vi "Wheel Set.vi"(9 "MotorControlDevRef":T2={"DeviceStatus"={"status"=FALSE, "code"=0, "source"=""}, "Type"=enum."PWM", "PWM"={"PWM Channel"=enum."Invalid", "DeadBand"={"Name"="", "maxPositivePwm"=0, "minPositivePwm"=0, "centerPwm"=0, "maxNegativePwm"=0, "minNegativePwm"=0, "angularRange"=0}}, "CAN"={"Device Number"=0, "Control Mode"=enum."Percent VBus", "Semaphore"=refnum, "Max Vout"=12.0, "TalonSRX Control Mode"=enum."Percent VBus"}, "Invert"=FALSE}, 10 "DevRef":string, 11 "Control Gains":T1={"Period (ms)"=20, "TBH Gain"=0.5, "Priority"=100, "PID gains"={"proportional gain (Kc)"=1.0, "integral time (Ti, min)"=0.01, "derivative time (Td, min)"=0.0}, "Stable (sec)"=20.0, "Range"=20.0} {"PID gains"."derivative time (Td, min)" format="%.3f"; "PID gains"."integral time (Ti, min)" format="%.3f"; "PID gains"."proportional gain (Kc)" format="%.3f"}) -> (0 "Error Out":errorcluster, 3 "Shooter Wheel DevRef Out":T9={"Shooter Config reference"=refnum, "Shooter Data"={"MotorControlDevRef"={"DeviceStatus"={"status"=FALSE, "code"=0, "source"=""}, "Type"=enum."PWM", "PWM"={"PWM Channel"=enum."Invalid", "DeadBand"={"Name"="", "maxPositivePwm"=0, "minPositivePwm"=0, "centerPwm"=0, "maxNegativePwm"=0, "minNegativePwm"=0, "angularRange"=0}}, "CAN"={"Device Number"=0, "Control Mode"=enum."Percent VBus", "Semaphore"=refnum, "Max Vout"=12.0, "TalonSRX Control Mode"=enum."Percent VBus"}, "Invert"=FALSE}, "Set Point"=refnum, "Actual"=refnum}})   [LabVIEW 2015, in "Wheel.lvlib"]
doc: "Help by FRC Team 836 - The RoboBees\n\nThis VI will set the desired Revolutions Per Minute (RPM) for a wheel."
uses:
  <userlib>/836-Library/Motion_Control/Shooter_Wheel/Wheel.lvlib
  <userlib>/836-Library/Motion_Control/Shooter_Wheel/WheelControl.ctl
  <userlib>/836-Library/Motion_Control/Shooter_Wheel/Config.ctl
  <userlib>/836-Library/Motion_Control/Shooter_Wheel/Data.ctl
  <vilib>/Rock Robotics/WPI/MotorControl/WPI_MotorControlDeviceRef.ctl
  <vilib>/Rock Robotics/WPI/MotorControl/WPI_MotorControlType.ctl
  <vilib>/Rock Robotics/SystemInterfaces/DIO/FPGA_DIOPWMChannel.ctl
  <vilib>/Rock Robotics/WPI/PWM/WPI_PWMDeadband.ctl
  <vilib>/Rock Robotics/WPI/CAN/Jaguar/SubVIs/WPI_CANJaguar_ControlMode.ctl
  <vilib>/Rock Robotics/WPI/CAN/TalonSRX/WPI_CANTalonSRX_APIControlMode.ctl
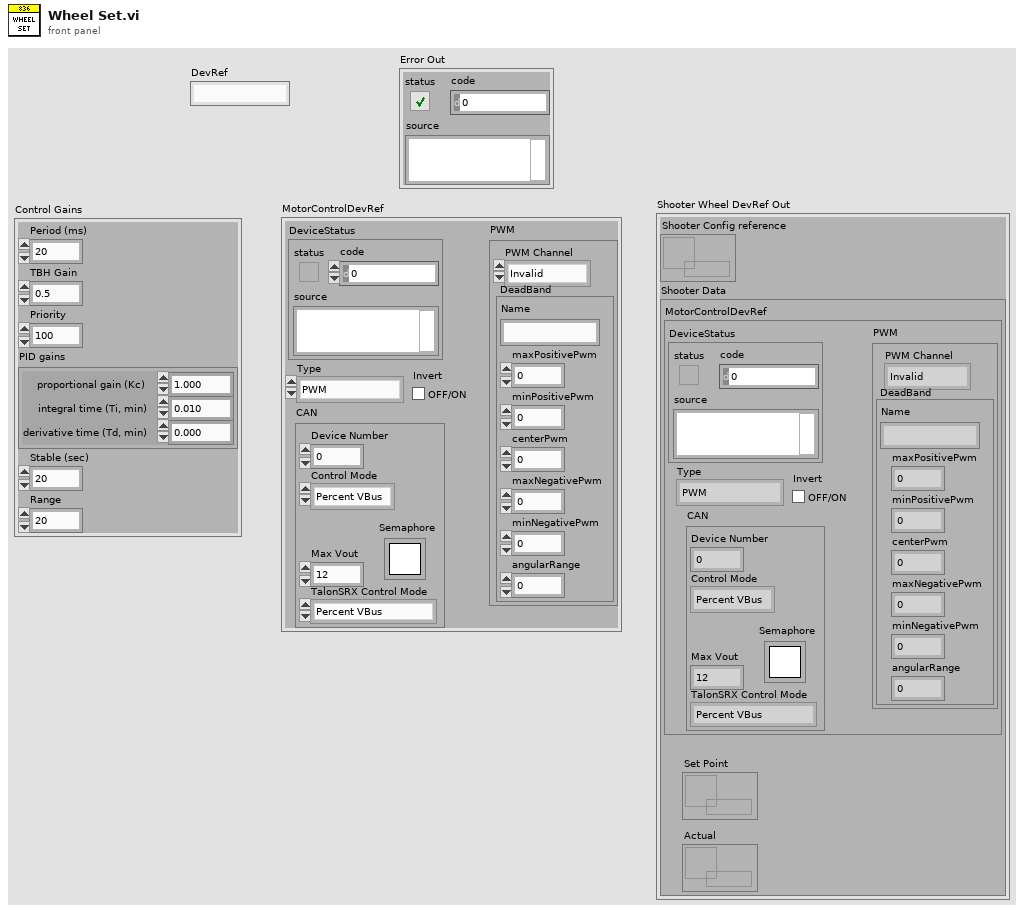
[diagram p1: front panel]
types:
  T1 = typedef "Wheel.lvlib/Config.ctl" = cluster{"Period (ms)":i64, "TBH Gain":dbl, "Priority":i32, "PID gains":cluster{"proportional gain (Kc)":dbl, "integral time (Ti, min)":dbl, "derivative time (Td, min)":dbl}, "Stable (sec)":dbl, "Range":dbl}
  T2 = typedef "WPI_MotorControlDeviceRef.ctl" = cluster{"DeviceStatus":errorcluster, "Type":T3, "PWM":cluster{"PWM Channel":T4, "DeadBand":T5}, "CAN":cluster{"Device Number":u8, "Control Mode":T6, "Semaphore":T7, "Max Vout":dbl, "TalonSRX Control Mode":T8}, "Invert":bool}
  T3 = typedef "WPI_MotorControlType.ctl" = enum16{"PWM", "CAN", "CANTalonSRX"}
  T4 = typedef "FPGA_DIOPWMChannel.ctl" = enum8{"PWM 0", "PWM 1", "PWM 2", "PWM 3", "PWM 4", "PWM 5", "PWM 6", "PWM 7", "PWM 8", "PWM 9", "PWM MXP 0", "PWM MXP 1", "PWM MXP 2", "PWM MXP 3", "PWM MXP 4", "PWM MXP 5", "PWM MXP 6", "PWM MXP 7", "PWM MXP 8", "PWM MXP 9", "Invalid"}
  T5 = typedef "WPI_PWMDeadband.ctl" = cluster{"Name":string, "maxPositivePwm":i32, "minPositivePwm":i32, "centerPwm":i32, "maxNegativePwm":i32, "minNegativePwm":i32, "angularRange":u16}
  T6 = typedef "WPI_CANJaguar_ControlMode.ctl" = enum8{"Percent VBus", "Current", "Speed", "Position", "Voltage"}
  T7 = typedef "Semaphore RefNum" = refnum<k1>
  T8 = typedef "WPI_CANTalonSRX_APIControlMode.ctl" = enum8{"Percent VBus", "Speed", "Position", "Slave", "Unchanged / Invalid", "Voltage Compensation", "Current", "Motion Profile"}
  T9 = typedef "Wheel.lvlib/WheelControl.ctl" = cluster{"Shooter Config reference":refnum<data-value>, "Shooter Data":T10}
  T10 = typedef "Wheel.lvlib/Data.ctl" = cluster{"MotorControlDevRef":T2, "Set Point":refnum<k33>, "Actual":refnum<k33>}
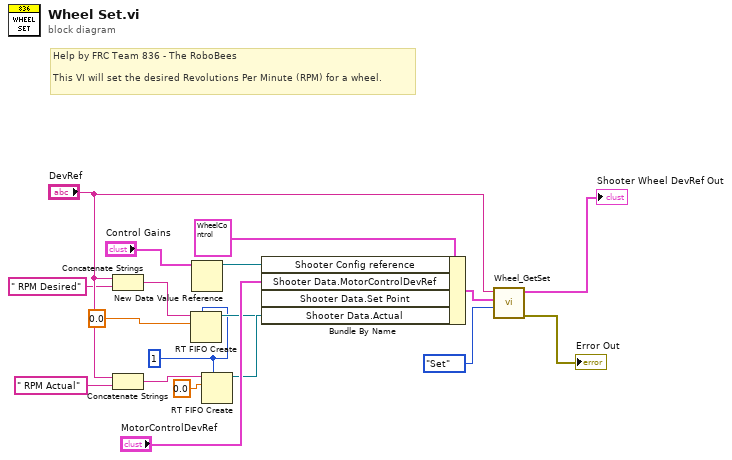
[diagram p0: block diagram]
diagram:
  w5 = u32 1 ("size (10)")
  # "Help by FRC Team 836 - The RoboBees\n\nThis VI will set the desired Revolutions Per Minute (RPM) for a wheel."
  n1 = Concatenate Strings("DevRef", " RPM Desired" ("string")) -> (w6:string)
  n2 = Concatenate Strings("DevRef", " RPM Actual" ("string")) -> (w4:string)
  n3 = RT FIFO Create(0:w6, 1:0.0 ("x"), 4:w5) -> (8:w8:refnum<k33>)  [unwired: 5 in, 2 out]
  n4 = New Data Value Reference(data value="Control Gains") -> (data value reference=w7:refnum<data-value>)  [unwired: 1 in, 1 out]
  n5 = RT FIFO Create(0:w4, 1:0.0, 4:w5) -> (8:w9:refnum<k33>)  [unwired: 5 in, 2 out]
  n6 = Bundle By Name(cluster=T9 {"Shooter Config reference"=refnum, "Shooter Data"={"MotorControlDevRef"={"DeviceStatus"={"status"=FALSE, "code"=0, "source"=""}, "Type"=enum."PWM", "PWM"={"PWM Channel"=enum."Invalid", "DeadBand"={"Name"="", "maxPositivePwm"=0, "minPositivePwm"=0, "centerPwm"=0, "maxNegativePwm"=0, "minNegativePwm"=0, "angularRange"=0}}, "CAN"={"Device Number"=0, "Control Mode"=enum."Percent VBus", "Semaphore"=refnum, "Max Vout"=12.0, "TalonSRX Control Mode"=enum."Percent VBus"}, "Invert"=FALSE}, "Set Point"=refnum, "Actual"=refnum}}, "Shooter Config reference"=w7, "Shooter Data.MotorControlDevRef"="MotorControlDevRef", "Shooter Data.Set Point"=w8, "Shooter Data.Actual"=w9) -> (w14:T9)
  n7 = call <userlib>:"Wheel_GetSet.vi"("Enum"=enum16{"Set", "Get"}."Set", "Shooter Wheel DevRef In"=w14, "DevRef"="DevRef") -> ("Error Out"=→"Error Out":errorcluster, "Shooter Wheel DevRef Out"=→"Shooter Wheel DevRef Out":T9)  [unwired: 7 in]
